vi "stable_for_time.vi"(1 "time (0 ms)":i32, 2 "Data":variant, 4 "Reset":bool caption="Reset (F)") -> (7 "stable for time?":bool)   [LabVIEW 2015]
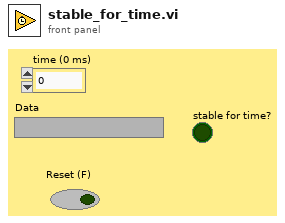
[diagram p1: front panel]
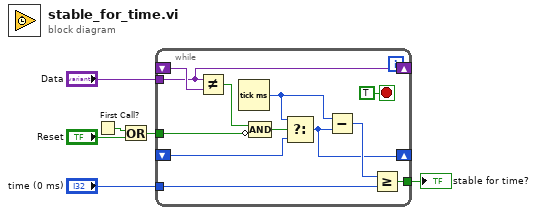
[diagram p0: block diagram]
diagram:
  n1 = First Call?() -> (First Call?: T/F=w5:bool)
  n2 = Or(x=w5, y="Reset") -> (x .or. y?=w3:bool)
  n3 = while {
    tunnel: "Data" -> [w8]
    tunnel: w3 -> [w12]
    tunnel: "time (0 ms)" -> [w18]
    tunnel: [w17] -> w1
    shift-right: [w8] -> _
    shift-left: _ -> [w16]
    shift-right: [w10] -> _
    shift-left: _ -> [w15]
    stop <- TRUE stop-if-true
    n4 = Not Equal?(x=w8, y=w16) -> (x != y?=w9:bool)
    n5 = Tick Count (ms) ("Now")() -> (millisecond timer value=w14:u32)
    n6 = Compound Arithmetic op=AND(w9, invert w12) -> (w11:bool)
    n7 = Select(t=w14, s=w11, f=w15) -> (s? t:f=w10:u32)
    n8 = Subtract(x=w14, y=w10) -> (x-y=w13:u32)
    n9 = Greater Or Equal?(x=w13, y=w18) -> (x >= y?=w17:bool)
  }
  "stable for time?" <- w1
